vi "readFromXML.vi"(8 "error in (no error)":errorcluster, 10 "XML in":string, 11 "CommandsForRotatorAxis in":refnum<class "CommandsForRotatorAxis.lvclass">) -> (0 "error out":errorcluster, 3 "CommandsForRotatorAxis out":refnum<class "CommandsForRotatorAxis.lvclass">)   [LabVIEW 2022 SP3, in "TCSDataDefinitions.lvlib" / "TCSMountControlCommand.lvlib" / "CommandsForRotatorAxis.lvlib" / "CommandsForRotatorAxis.lvclass"]
uses:
  CommandsForRotatorAxis.lvclass
  TCSMCCCommand/TCSMCCCommand.lvclass
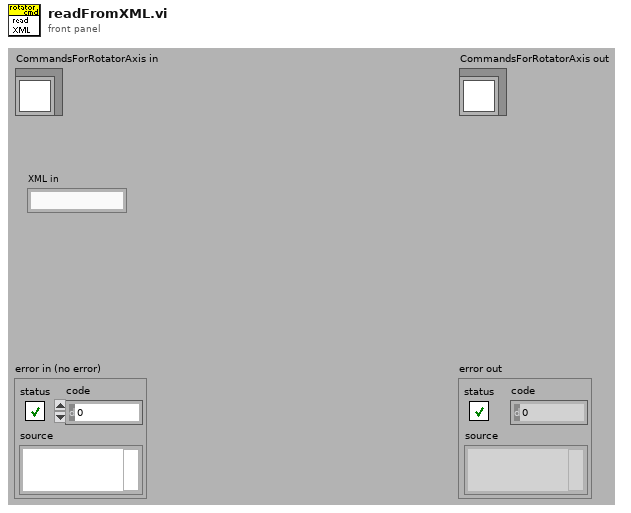
[diagram p1: front panel]
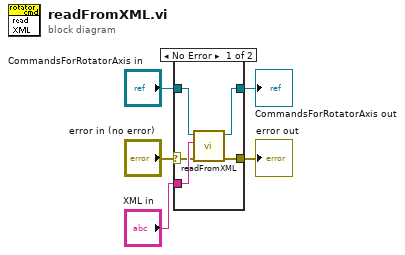
[diagram p0: block diagram]
diagram:
  n1 = case shown="No Error" "error in (no error)" {
    selector: "error in (no error)" -> [w9 w12]
    tunnel: [w6 w12] -> w4
    tunnel: [w7 w11] -> w2
    tunnel: "CommandsForRotatorAxis in" -> [w8 w11]
    tunnel: "XML in" -> [w10 _]
    frame No Error {
      n2 = call-parent "readFromXML.vi"("error in (no error)"=w9, "XML in"=w10, "TCSMCCCommand in"=w8) -> ("error out"=w6:errorcluster, "TCSMCCCommand out"=w7:refnum<class "CommandsForRotatorAxis.lvclass">)  [unwired: 7 out]
    }
    frame Error {
    }
  }
  "error out" <- w4
  "CommandsForRotatorAxis out" <- w2
